vi "DAQ.Init.vi"(8 "error in (no error)":errorcluster, 11 "DAQmx.AO in":refnum<class "DAQmx.AO.lvclass">) -> (0 "error out":errorcluster, 3 "DAQmx.AO out":refnum<class "DAQmx.AO.lvclass">)   [LabVIEW 2016, in "DAQmx.AO.lvclass"]
uses:
  DAQmx.AO.lvclass
  C:/user/patrick/hg/lockin.SMO/lvsrc/DAQ/DAQ.lvclass
  C:/user/patrick/hg/lockin.SMO/lvsrc/DAQmx/DAQmx.lvclass
  DAQ/DAQ.lvclass/DAQ.ctl
  DAQmx.AO.lvclass/DAQmx.AO.ctl
  DAQmx/DAQmx.lvclass/DAQmx.ctl
  <vilib>/DAQmx/create/channels.llb/DAQmx Create Channel (AO-Voltage-Basic).vi
  <vilib>/DAQmx/configure/timing.llb/DAQmx Timing (Sample Clock).vi
  <resource>/objmgr/daqmx.rc
  DAQ/DAQ.lvclass
  DAQmx/DAQmx.lvclass
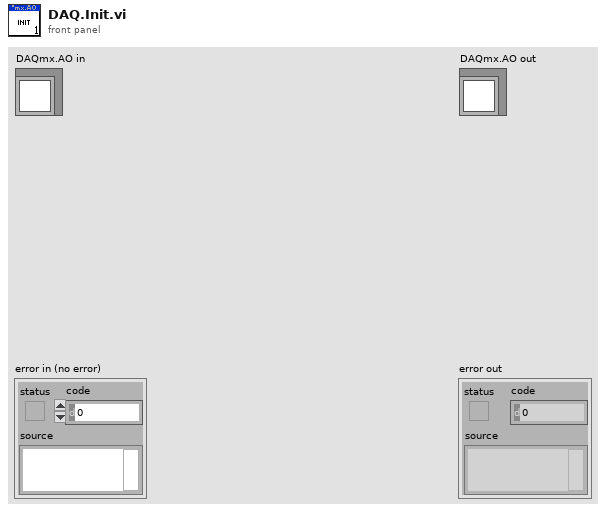
[diagram p1: front panel]
types:
  T1 = typedef "DAQ.lvclass/DAQ.Config.ctl" = cluster{"Channels":T2, "DAQType":T3, "minimum value":dbl, "maximum value":dbl, "sampling info":T4, "SamplingMode":T5}
  T2 = typedef "PrivateEvents--DAQ.AI.Channels.ctl" = string
  T3 = typedef "DAQ.lvclass/DAQType.ctl" = enum16{"AI", "AO"}
  T4 = typedef "DAQ.lvclass/SamplingInfo.ctl" = cluster{"Fs":dbl, "#s":dbl}
  T5 = typedef "DAQ.lvclass/SamplingMode.ctl" = enum16{"Continuous", "Finite"}
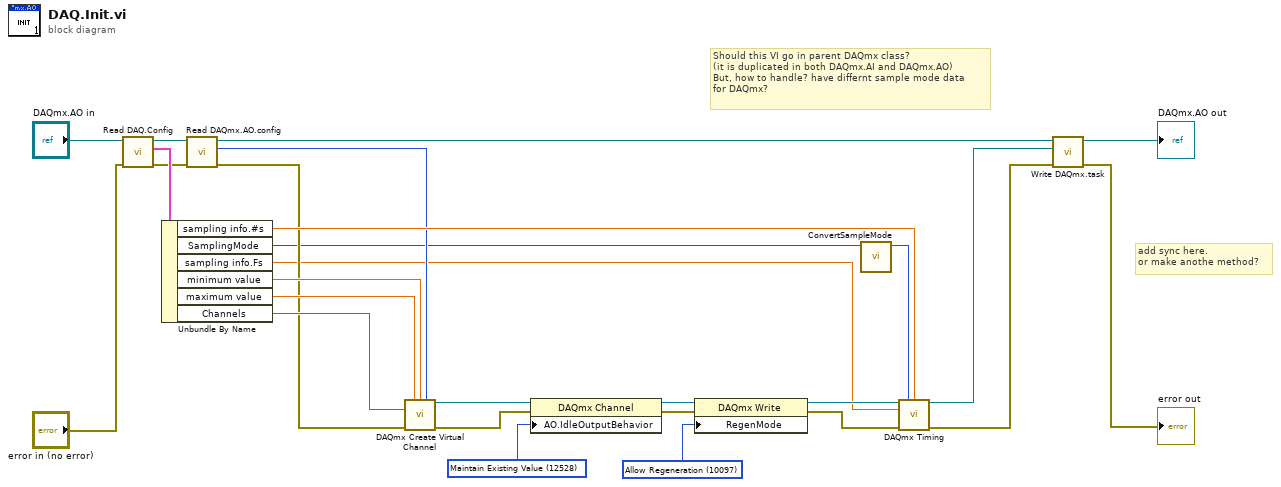
[diagram p0: block diagram]
diagram:
  w26 = 10097 items=["Allow Regeneration"=10097, "Do Not Allow Regeneration"=10158] ("RegenMode")
  w27 = 12528 items=["Zero Volts"=12526, "High-Impedance"=12527, "Maintain Existing Value"=12528] ("AO.IdleOutputBehavior")
  # "Should this VI go in parent DAQmx class?\n(it is duplicated in both DAQmx.AI and DAQmx.AO)\nBut, how to handle? have differnt sample mode data\nfor DAQmx?"
  # "add sync here.\nor make anothe method?"
  n1 = call "Read DAQ.Config.vi"("error in (no error)"="error in (no error)", "DAQ in"="DAQmx.AO in") -> ("error out"=w7:errorcluster, "Configuration"=w18:T1, "DAQ out"=w8:refnum<class "DAQmx.AO.lvclass">)  [unwired: 7 in]
  n2 = Unbundle By Name(w18) -> ("sampling info.#s"=w14:dbl, "SamplingMode"=w3:T5, "sampling info.Fs"=w1:dbl, "minimum value"=w17:dbl, "maximum value"=w16:dbl, "Channels"=w15:T2)
  n3 = call "Read DAQmx.AO.config.vi"("error in (no error)"=w7, "DAQmx.AO in"=w8) -> ("error out"=w4:errorcluster, "output terminal configuration"=w6:i32, "DAQmx.AO out"=w5:refnum<class "DAQmx.AO.lvclass">)  [unwired: 7 in]
  n4 = call-poly <vilib>:"DAQmx Create Virtual Channel.vi"("maximum value"=w16, "minimum value"=w17, "output terminal configuration"=w6, "physical channels"=w15, "error in"=w4) -> ("task out"=w23:refnum<k21>, "error out"=w22:errorcluster)  [unwired: 9 in]
  n5 = property class="DAQmx Channel"(reference=w23, error in=w22, "AO.IdleOutputBehavior"=w27) -> (reference out=w21:refnum<k21>, error out=w20:errorcluster)
  n6 = property class="DAQmx Write"(reference=w21, error in=w20, "RegenMode"=w26) -> (reference out=w25:refnum<k21>, error out=w24:errorcluster)
  n7 = call "ConvertSampleMode.vi"("SamplingMode"=w3) -> ("sample mode"=w2:i32)  [unwired: 10 in]
  n8 = call-poly <vilib>:"DAQmx Timing.vi"("task/channels in"=w25, "sample mode"=w2, "samples per channel"=w14, "rate"=w1, "error in"=w24) -> ("task out"=w12:refnum<k21>, "error out"=w11:errorcluster)  [unwired: 9 in]
  n9 = call "Write DAQmx.task.vi"("error in (no error)"=w11, "task"=w12, "DAQmx in"=w5) -> ("error out"=→"error out":errorcluster, "DAQmx out"=→"DAQmx.AO out":refnum<class "DAQmx.AO.lvclass">)  [unwired: 7 in]
